vi "Emballage calcule nb ds carton.vi"(2 "Tableau \nlots OUT":string[][](array[string])=[["0801", "13"], ["0802", "27"], ["0803", "31"]], 4 "Quantité de la cmde":i32) -> (0 "Tab n° carton - nb ds carton":i32[][](array[numeric]), 1 "Nb total cartons":i32)   [LabVIEW 2020]
doc: "Calcule le nombre de carton attendu ainsi que le nb de valves dans chaque carton selon que l'om peut mélanger les lots ou non, le nb de lots différents le cas échéant, la quantité de la commande et le nb de valves par carton."
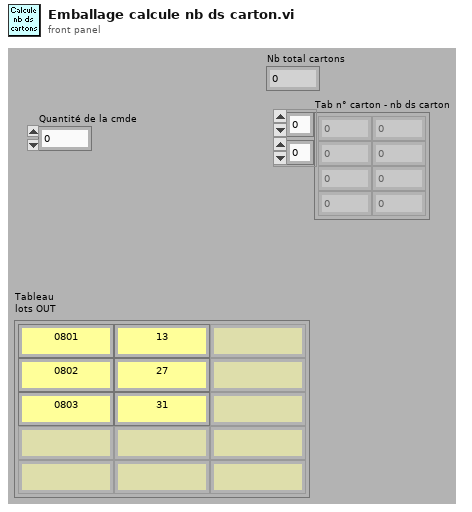
[diagram p1: front panel]
types:
  T1 = typedef "Emballage_BDD_param_Produit.ctl" = cluster{"No_Valve_FAS":string, "suffixe":string, "designation":string, "indice_produit":string, "code_barre_fixe":string, "affiche_code_barre_client":string, "affiche_no_client":string, "Nb_vlve_par_carton":u16, "melange_des_lots_possible":string, "id_article":string, "Indice_Rev":string, "Famille":string, "date":string, "code_barre_fixe_Fin":string, "Longeur_No_Serie":string}
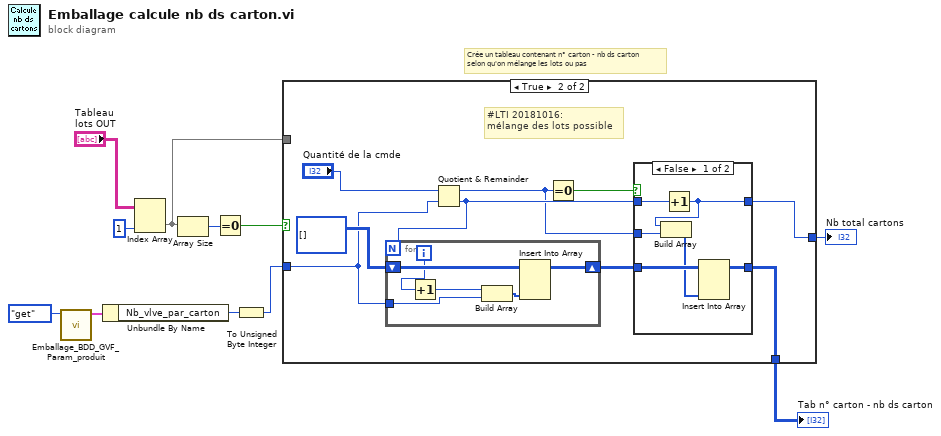
[diagram p0: block diagram]
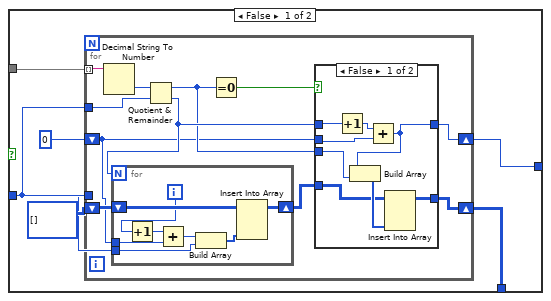
[diagram p2: hidden frame]
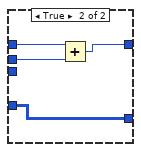
[diagram p3: hidden frame]
diagram:
  # "Crée un tableau contenant n° carton - nb ds carton\nselon qu'on mélange les lots ou pas"
  n1 = call "Emballage_BDD_GVF_Param_produit.vi"("Énum"=enum16{"set", "get"}."get") -> ("CLS_param_produit"=w4:T1)  [unwired: 7 in, 3 out]
  n2 = Unbundle By Name(w4) -> ("Nb_vlve_par_carton"=w3:u16)
  n3 = Index Array(array="Tableau \nlots OUT", index (col)=1 ("indice désactivé (col)")) -> (element=w7:string[])  [unwired: 1 in]
  n4 = Array Size(array=w7) -> (size(s)=w10:i32)
  n5 = Equal To 0?(x=w10) -> (x = 0?=w9:bool)
  n6 = To Unsigned Byte Integer(number=w3) -> (unsigned 8bit integer=w2:u8)
  n7 = case shown="True" w9 {
    tunnel: [w16 w57] -> w6
    tunnel: w2 -> [w14 w53]
    tunnel: w7 -> [w17 _]
    tunnel: [w13 w50] -> w5
    frame False {
      n8 = for {
        tunnel: w17 -> [w27] mode=indexing
        tunnel: w14 -> [w28]
        shift-right: [w25] -> w16
        shift-left: 0 -> [w18]
        tunnel: w14 -> [w23]
        shift-right: [w20] -> w13
        shift-left: i32[][] [] -> [w19]
        n9 = Decimal String To Number(string=w27) -> (number=w26:i32)  [unwired: 2 in, 1 out]
        n10 = Quotient & Remainder(x=w26, y=w28) -> (x-y*floor(x/y)=w21:i32, floor(x/y)=w24:i32)
        n11 = for {
          N: w24 -> [_]
          tunnel: w23 -> [w34]
          shift-right: [w36] -> w22
          shift-left: w19 -> [w37]
          tunnel: w18 -> [w31]
          i -> [w35]
          n12 = Increment(x=w35) -> (x+1=w32:i32)
          n13 = Add(x=w32, y=w31) -> (x+y=w30:i32)
          n14 = Build Array(w30, w34) -> (w33:i32[])
          n15 = Insert Into Array(array=w37, new element=w33) -> (w36:i32[][])  [unwired: 2 in]
        }
        n16 = Equal To 0?(x=w21) -> (x = 0?=w29:bool)
        n17 = case shown="False" w29 {
          tunnel: w24 -> [w45 w49]
          tunnel: [w39 w47] -> w25
          tunnel: w18 -> [w44 w48]
          tunnel: w22 -> [w41 w46]
          tunnel: w21 -> [w40 _]
          tunnel: [w38 w46] -> w20
          frame False {
            n18 = Increment(x=w45) -> (x+1=w43:i32)
            n19 = Add(x=w43, y=w44) -> (x+y=w39:i32)
            n20 = Build Array(w39, w40) -> (w42:i32[])
            n21 = Insert Into Array(array=w41, new element=w42) -> (w38:i32[][])  [unwired: 2 in]
          }
          frame True {
            n22 = Add(x=w49, y=w48) -> (x+y=w47:i32)
          }
        }
      }
    }
    frame True {
      # "#LTI 20181016:\nmélange des lots possible"
      n23 = Quotient & Remainder(x="Quantité de la cmde", y=w53) -> (x-y*floor(x/y)=w51:i32, floor(x/y)=w55:i32)
      n24 = for {
        N: w55 -> [_]
        tunnel: w53 -> [w61]
        shift-right: [w63] -> w52
        shift-left: i32[][] [] -> [w64]
        i -> [w62]
        n25 = Increment(x=w62) -> (x+1=w59:i32)
        n26 = Build Array(w59, w61) -> (w60:i32[])
        n27 = Insert Into Array(array=w64, new element=w60) -> (w63:i32[][])  [unwired: 2 in]
      }
      n28 = Equal To 0?(x=w51) -> (x = 0?=w58:bool)
      n29 = case shown="False" w58 {
        tunnel: w55 -> [w70 w72]
        tunnel: [w67 w72] -> w57
        tunnel: w52 -> [w69 w71]
        tunnel: [w68 w71] -> w50
        tunnel: w51 -> [w66 _]
        frame False {
          n30 = Increment(x=w70) -> (x+1=w67:i32)
          n31 = Build Array(w67, w66) -> (w65:i32[])
          n32 = Insert Into Array(array=w69, new element=w65) -> (w68:i32[][])  [unwired: 2 in]
        }
        frame True {
        }
      }
    }
  }
  "Nb total cartons" <- w6
  "Tab n° carton - nb ds carton" <- w5
